vi "Jump_UiVi.vi"(4 "reference":refnum<vi>) -> ()   [LabVIEW 2021]
panel:
  in  "error in (no error)":errorcluster
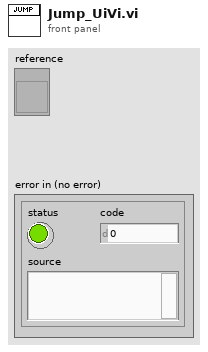
[diagram p1: front panel]
types:
  T1 = enum32{"Invalid", "Standard", "Closed", "Hidden", "Minimized", "Maximized"}
  T2 = enum32{"Bad", "Idle", "Run top level", "Running"}
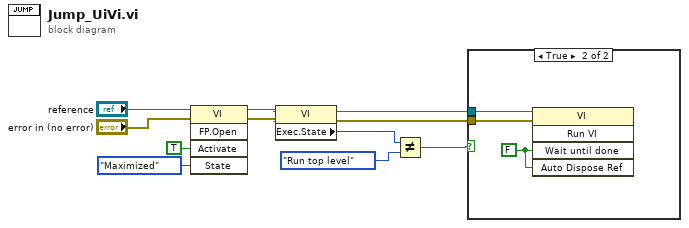
[diagram p0: block diagram]
diagram:
  n1 = invoke class="VI" method="FP.Open"(reference="reference", error in="error in (no error)", "Activate"=TRUE ("Activate?"), "State"=T1."Maximized") -> (reference out=w11:refnum<vi>, error out=w10:errorcluster)  [unwired: 1 in, 3 out]
  n2 = property class="VI"(reference=w11, error in=w10) -> (reference out=w7:refnum<vi>, error out=w6:errorcluster, "Exec.State"=w4:T2)
  n3 = Not Equal?(x=w4, y=T2."Run top level") -> (x != y?=w5:bool)
  n4 = case shown="True" w5 {
    tunnel: w7 -> [_ w14]
    tunnel: w6 -> [_ w13]
    frame False {
    }
    frame True {
      w12 = FALSE ("Wait Until Done")
      n5 = invoke class="VI" method="Run VI"(reference=w14, error in=w13, "Wait until done"=w12, "Auto Dispose Ref"=w12) -> ()  [unwired: 1 in, 5 out]
    }
  }
